vi "Define Parameter.vi"(8 "error in (no error)":errorcluster, 11 "Analyze Total Counts in":refnum<class "Analyze Total Counts.lvclass">) -> (0 "error out":errorcluster, 3 "Analyze Total Counts out":refnum<class "Analyze Total Counts.lvclass">)   [LabVIEW 2014, in "Analyze.lvlib" / "Analyze BaseClass.lvlib" / "Analyze Total Counts.lvclass"]
uses:
  Analyze Total Counts.lvclass
  Analyze BaseClass/Analyze BaseClass/Analyze BaseClass.lvclass
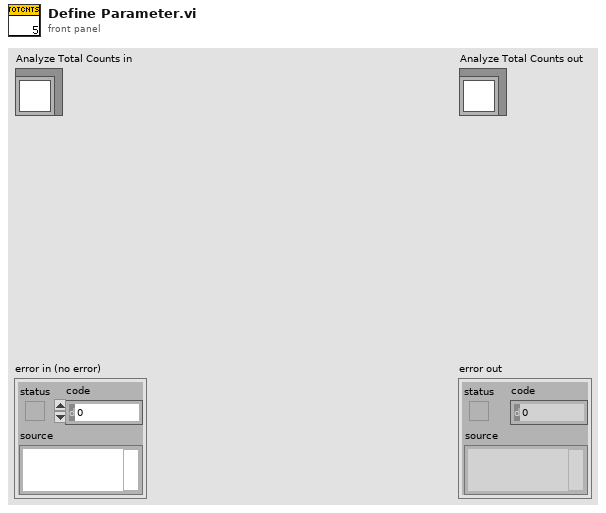
[diagram p1: front panel]
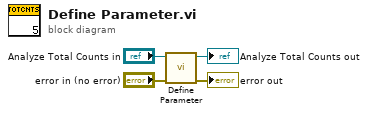
[diagram p0: block diagram]
diagram:
  n1 = call-parent "Define Parameter.vi"("error in (no error)"="error in (no error)", "Analyze BaseClass in"="Analyze Total Counts in") -> ("error out"=→"error out":errorcluster, "Analyze BaseClass out"=→"Analyze Total Counts out":refnum<class "Analyze Total Counts.lvclass">)  [unwired: 8 in]
